vi "test Add and Get Timing Channels.vi"(8 "error in":errorcluster, 11 "TestCase in":refnum<class "Scripting.lvclass">) -> (0 "error out":errorcluster)   [LabVIEW 2020, in "Scripting.lvclass"]
uses:
  Scripting.lvclass
  Scripting.lvclass/Scripting.ctl
  <vilib>/addons/_JKI Toolkits/VI Tester/TestCase.llb/TestCase.lvclass
  Scripting/Ballard/Ballard ARINC 429 Scripting.lvlib
  C:/Program Files (x86)/National Instruments/LabVIEW 2020/vi.lib/addons/_JKI Toolkits/VI Tester/TestCase.llb/TestCase.lvclass
panel:
  out "TestCase out":refnum<class "Scripting.lvclass">
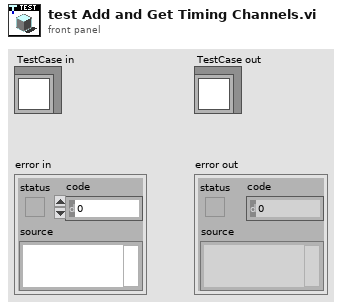
[diagram p1: front panel]
types:
  T1 = typedef "Custom Device API.lvlib/Custom Device Item Ref.ctl" = u64
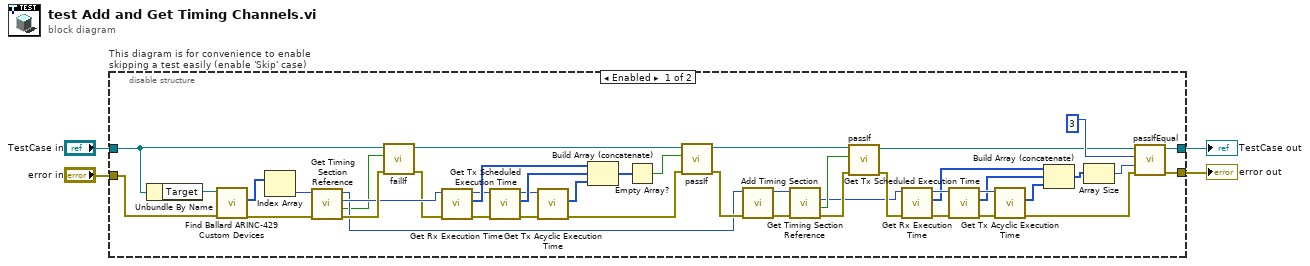
[diagram p0: block diagram]
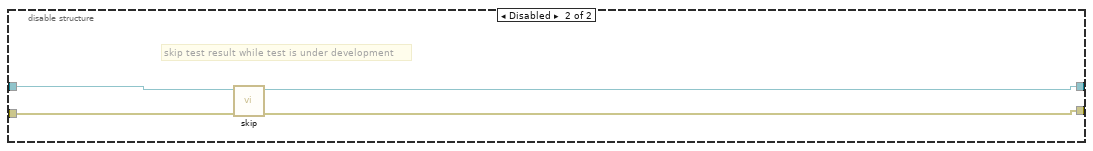
[diagram p2: hidden frame]
diagram:
  n1 = disable-structure "This diagram is for convenience to enable skipping a test easily (enable 'Skip' case)" shown="Enabled" {
    disable-tunnel: "TestCase in" -> [w48 w52]
    disable-tunnel: [w15 w50] -> w1
    disable-tunnel: [w16 w51] -> w3
    disable-tunnel: "error in" -> [w46 w49]
    frame Enabled {
      n2 = Unbundle By Name(w48) -> ("Target"=w47:refnum<k24>)
      n3 = call "Find Ballard ARINC-429 Custom Devices.vi"("error in"=w46, "target in"=w47) -> ("error out"=w43:errorcluster, "Ballard ARINC 429 custom devices"=w45:u64[])  [unwired: 7 in, 1 out]
      n4 = Index Array(array=w45) -> (element=w44:u64)  [unwired: 1 in]
      n5 = call "Get Timing Section Reference.vi"("error in"=w43, "Ballard ARINC 429 ref"=w44) -> ("error out"=w42:errorcluster, "found"=w14:bool, "timing section reference"=w37:T1, "Ballard ARINC 429 ref out"=w28:T1)  [unwired: 6 in]
      n6 = call-dynamic "failIf.vi"("error in (no error)"=w42, "fail"=w14, "TestCase in"=w48) -> ("error out"=w7:errorcluster, "TestCase out"=w36:refnum<class "Scripting.lvclass">)  [unwired: 7 in]
      n7 = call "Get Rx Execution Time.vi"("error in"=w7, "timing section in"=w37) -> ("error out"=w39:errorcluster, "rx execution time ref"=w34:T1[], "timing section out"=w21:T1)  [unwired: 7 in]
      n8 = call "Get Tx Scheduled Execution Time.vi"("error in"=w39, "timing section in"=w21) -> ("error out"=w38:errorcluster, "tx scheduled execution time ref"=w33:T1[], "timing section out"=w20:T1)  [unwired: 7 in]
      n9 = call "Get Tx Acyclic Execution Time.vi"("error in"=w38, "timing section in"=w20) -> ("error out"=w35:errorcluster, "tx acyclic execution time ref"=w32:T1[])  [unwired: 7 in, 1 out]
      n10 = Build Array (concatenate)(w34, w33, w32) -> (w31:T1[])
      n11 = Empty Array?(array=w31) -> (empty?=w30:bool)
      n12 = call-dynamic "passIf.vi"("error in (no error)"=w35, "pass"=w30, "TestCase in"=w36) -> ("error out"=w29:errorcluster, "TestCase out"=w27:refnum<class "Scripting.lvclass">)  [unwired: 7 in]
      n13 = call "Add Timing Section.vi"("error in"=w29, "custom device ref"=w28) -> ("error out"=w41:errorcluster, "custom device ref out"=w40:T1)  [unwired: 7 in, 1 out]
      n14 = call "Get Timing Section Reference.vi"("error in"=w41, "Ballard ARINC 429 ref"=w40) -> ("error out"=w25:errorcluster, "found"=w13:bool, "timing section reference"=w5:T1)  [unwired: 6 in, 1 out]
      n15 = call-dynamic "passIf.vi"("error in (no error)"=w25, "pass"=w13, "TestCase in"=w27) -> ("error out"=w6:errorcluster, "TestCase out"=w9:refnum<class "Scripting.lvclass">)  [unwired: 7 in]
      n16 = call "Get Rx Execution Time.vi"("error in"=w6, "timing section in"=w5) -> ("error out"=w26:errorcluster, "rx execution time ref"=w19:T1[], "timing section out"=w23:T1)  [unwired: 7 in]
      n17 = call "Get Tx Scheduled Execution Time.vi"("error in"=w26, "timing section in"=w23) -> ("error out"=w24:errorcluster, "tx scheduled execution time ref"=w18:T1[], "timing section out"=w22:T1)  [unwired: 7 in]
      n18 = call "Get Tx Acyclic Execution Time.vi"("error in"=w24, "timing section in"=w22) -> ("error out"=w8:errorcluster, "tx acyclic execution time ref"=w17:T1[])  [unwired: 7 in, 1 out]
      n19 = Build Array (concatenate)(w19, w18, w17) -> (w12:T1[])
      n20 = Array Size(array=w12) -> (size(s)=w11:i32)
      n21 = call-dynamic "passIfEqual.vi"("error in (no error)"=w8, "y"=w11, "x"=3, "TestCase in"=w9) -> ("error out"=w16:errorcluster, "TestCase out"=w15:refnum<class "Scripting.lvclass">)  [unwired: 6 in]
    }
    frame Disabled {
      # "skip test result while test is under development"
      n22 = call <vilib>:"skip.vi"("error in (no error)"=w49, "TestCase in"=w52) -> ("error out"=w51:errorcluster, "TestCase out"=w50:refnum<class "Scripting.lvclass">)  [unwired: 8 in]
    }
  }
  "error out" <- w3
  "TestCase out" <- w1
